vi "Arduino_LabView.vi"() -> ()   [LabVIEW 2019]
uses:
  <vilib>/Instr/_visa.llb/VISA Configure Serial Port (Instr).vi
panel:
  in  "COM":refnum<visa-resource-name>
  out "read buffer":string
  in  "stop":bool
  out "Meter":dbl(knob) scale=0.0..24.0
  out "Gauge":dbl(knob) scale=0.0..180.0
  out "Tank":dbl(slide) scale=0.0..100.0
  out "Thermometer":dbl(slide) scale=0.0..50.0
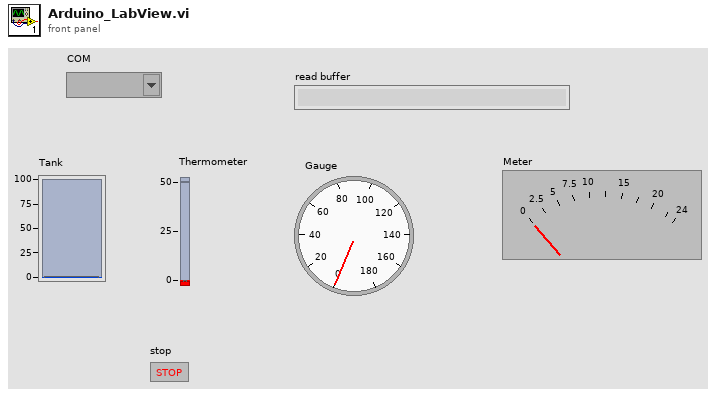
[diagram p1: front panel]
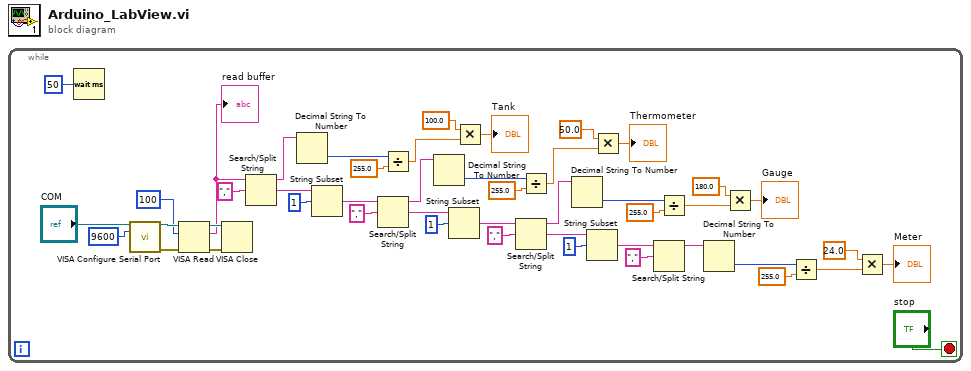
[diagram p0: block diagram]
diagram:
  n1 = while {
    stop <- "stop" stop-if-true
    n2 = Wait (ms)(milliseconds to wait=u32 50) -> ()  [unwired: 1 out]
    n3 = call-poly "VISA Configure Serial Port"("VISA resource name"="COM", "baud rate (9600)"=u32 9600) -> ("VISA resource name out"=w44:refnum<visa-resource-name>, "error out"=w45:errorcluster)  [unwired: 12 in]
    n4 = VISA Read(VISA resource name=w44, byte count=u32 100, error in (no error)=w45) -> (VISA resource name out=w41:refnum<visa-resource-name>, read buffer=w38:string, error out=w42:errorcluster)  [unwired: 1 out]
    "read buffer" <- w38
    n5 = VISA Close(VISA resource name=w41, error in (no error)=w42) -> ()  [unwired: 1 out]
    n6 = Search/Split String(string=w38, search string/char (-)=",") -> (substring before match=w36:string, match + rest of string=w23:string)  [unwired: 1 in, 1 out]
    n7 = Decimal String To Number(string=w36) -> (number=w31:i32)  [unwired: 2 in, 1 out]
    n8 = String Subset(string=w23, offset (0)=1) -> (substring=w22:string)  [unwired: 1 in]
    n9 = Search/Split String(string=w22, search string/char (-)=",") -> (substring before match=w29:string, match + rest of string=w11:string)  [unwired: 1 in, 1 out]
    n10 = Divide(x=w31, y=255.0) -> (x/y=w33:dbl)
    n11 = Decimal String To Number(string=w29) -> (number=w25:i32)  [unwired: 2 in, 1 out]
    n12 = String Subset(string=w11, offset (0)=1) -> (substring=w14:string)  [unwired: 1 in]
    n13 = Multiply(x=100.0, y=w33) -> (x*y=→"Tank":dbl)
    n14 = Search/Split String(string=w14, search string/char (-)=",") -> (substring before match=w19:string, match + rest of string=w2:string)  [unwired: 1 in, 1 out]
    n15 = Divide(x=w25, y=255.0) -> (x/y=w27:dbl)
    n16 = Decimal String To Number(string=w19) -> (number=w15:i32)  [unwired: 2 in, 1 out]
    n17 = String Subset(string=w2, offset (0)=1) -> (substring=w4:string)  [unwired: 1 in]
    n18 = Multiply(x=50.0, y=w27) -> (x*y=→"Thermometer":dbl)
    n19 = Search/Split String(string=w4, search string/char (-)=",") -> (substring before match=w9:string)  [unwired: 1 in, 2 out]
    n20 = Divide(x=w15, y=255.0) -> (x/y=w17:dbl)
    n21 = Decimal String To Number(string=w9) -> (number=w5:i32)  [unwired: 2 in, 1 out]
    n22 = Multiply(x=180.0, y=w17) -> (x*y=→"Gauge":dbl)
    n23 = Divide(x=w5, y=255.0) -> (x/y=w7:dbl)
    n24 = Multiply(x=24.0, y=w7) -> (x*y=→"Meter":dbl)
  }
